vi "Read configuration.vi"(8 "error in":errorcluster, 11 "Custom Temperature Controller editor node in":refnum<class "Custom Temperature Controller editor node.lvclass">) -> (0 "error out":errorcluster, 2 "configuration":refnum<class "NISE_CEF_serializable configuration.lvclass">, 3 "Custom Temperature Controller editor node out":refnum<class "Custom Temperature Controller editor node.lvclass">)   [LabVIEW 2021, in "Custom Temperature Controller editor node.lvclass"]
uses:
  Custom Temperature Controller editor node.lvclass
  <vilib>/NI/Configuration Framework/serializable configuration/NISE_CEF_serializable configuration.lvclass
  Custom Temperature Controller editor node.lvclass/Custom Temperature Controller editor node.ctl
  module/configuration/Custom Temperature Controller configuration.lvclass
  C:/Program Files (x86)/National Instruments/LabVIEW 2021/vi.lib/NI/Configuration Framework/serializable configuration/NISE_CEF_serializable configuration.lvclass
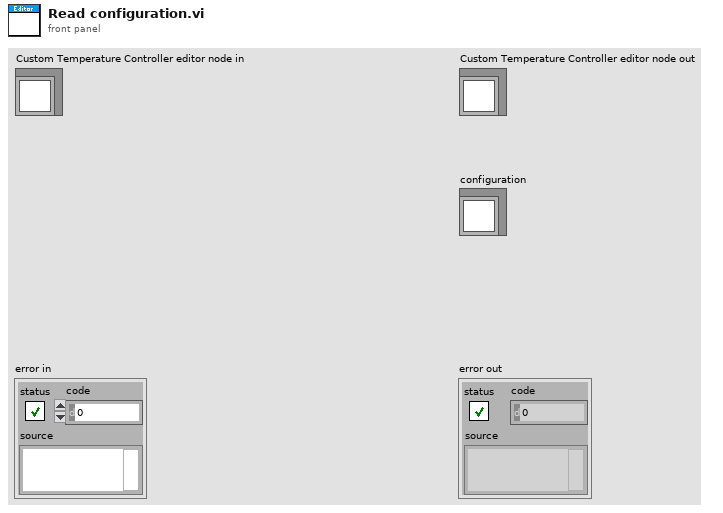
[diagram p1: front panel]
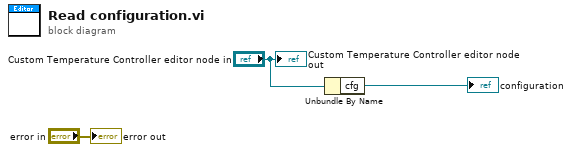
[diagram p0: block diagram]
diagram:
  n1 = Unbundle By Name("Custom Temperature Controller editor node in") -> ("cfg"=→"configuration":refnum<class "Custom Temperature Controller configuration.lvclass">)
  "error out" <- "error in"
  "Custom Temperature Controller editor node out" <- "Custom Temperature Controller editor node in"
